vi "Actor Core.vi"(8 "error in":errorcluster, 11 "Nested in":refnum<class "User Interface.lvclass">) -> (0 "error out":errorcluster, 3 "Actor out":refnum<class "Actor.lvclass">)   [LabVIEW 2022 SP3, in "User Interface.lvlib" / "User Interface.lvclass"]
doc: "(<B>Filename</B>: Actor Framework.lvlib:Actor.lvclass:Actor Core.vi)\n\nReceives messages to the actor, reacts to them, and initiates any error handling that may shut the actor down.\n\nDescendant classes may override this VI to append parallel tasks for the actor to complete while it handles messages. Overrides use the Call Parent Method node."
uses:
  User Interface.lvclass
  C:/Program Files/National Instruments/LabVIEW 2022/vi.lib/ActorFramework/Actor/Actor.lvclass
  <vilib>/ActorFramework/Actor/Actor.lvclass
  Typedefs/UI Helper Loop States.ctl
  User Interface.lvclass/User Interface.ctl
  <vilib>/ActorFramework/Actor/Actor.lvclass/Actor.ctl
  <vilib>/ActorFramework/Message Enqueuer/Message Enqueuer.lvclass/Message Enqueuer.ctl
  User Interface Messages/Update Status String Msg/Update Status String Msg.lvclass/Update Status String Msg.ctl
  User Interface Messages/Stop Test using Abs Msg/Stop Test using Abs Msg.lvclass/Stop Test using Abs Msg.ctl
  User Interface Messages/Generate Report Event using Abs Msg/Generate Report Event using Abs Msg.lvclass/Generate Report Event using Abs Msg.ctl
  <vilib>/Utility/miscctls.llb/LVRowAndColumnTypeDef.ctl
  User Interface Messages/Send Abs Start Test Msg/Start Test using Abs Msg.lvclass/Start Test using Abs Msg.ctl
  <vilib>/ActorFramework/Message Enqueuer/Init from Existing Queue.vi
  <vilib>/ActorFramework/Message Enqueuer/Enqueue.vi
  User Interface Messages/Close Application using Abs Msg/Close Application using Abs Msg.lvclass
  C:/Program Files/National Instruments/LabVIEW 2022/vi.lib/ActorFramework/Message/Message.lvclass
  User Interface Messages/Update Status String Msg/Update Status String Msg.lvclass
  User Interface Messages/Stop Test using Abs Msg/Stop Test using Abs Msg.lvclass
  User Interface Messages/Generate Report Event using Abs Msg/Generate Report Event using Abs Msg.lvclass
  User Interface Messages/Send Abs Start Test Msg/Start Test using Abs Msg.lvclass
  <vilib>/ActorFramework/Message Priority Queue/Priority Enqueue.vi
  <vilib>/ActorFramework/Message Enqueuer/Message Enqueuer.lvclass
  User Interface.lvlib
panel:
  in  "Logout":bool
  out "Machine":string
  out "User":string
  in  "Help":bool
  in  "Tab Control":enum32{"Test Execution", "Test Configuration"}(tab)
  in  "Load Selection":bool
  in  "Save Selection":bool
  in  "Overall Result":string
  in  "Print Report":bool
  in  "Stop Test":bool
  in  "Start Test":bool
  in  "Available Tests":i32[](listbox)
  in  "Test Configuration":T1(tab)
  in  "Ping Test":T2(array[cluster])
  in  "Select Path":path
  in  "Select a byte stream File Path":path
  in  "Select Test(s)":u16(ring)
  in  "Clear Status":bool
  out "Status":string
  # "Test Application v0.0"
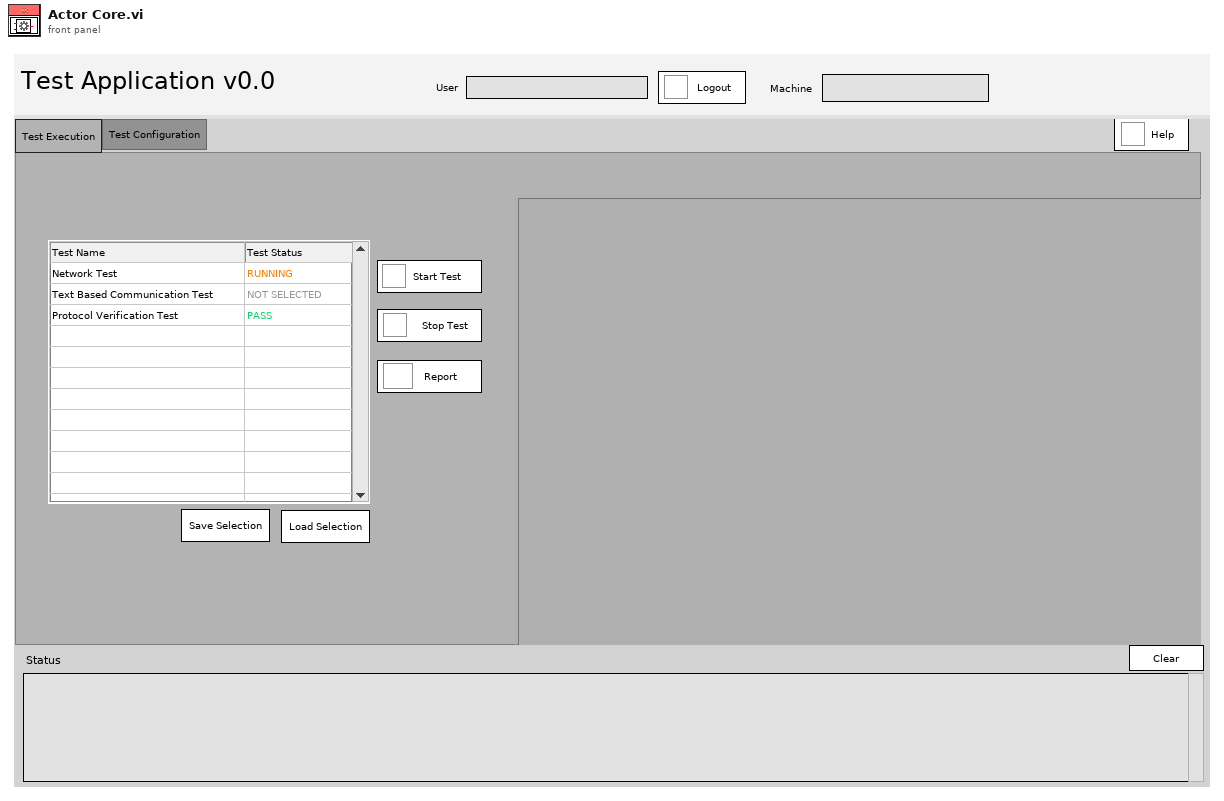
[diagram p1: front panel]
types:
  T1 = enum32{"None", "Network Test", "Text Based Communication Test", "Protocol Verification Test"}
  T2 = cluster{"IP/Address":string, "PacketSize":i32, "timeout":i32, "Packet Count":i32, "Min Expected Packed Return %":dbl, "Ping Result":cluster{"Result?":bool, "Actual Packet Return %":dbl}}[]
  T3 = typedef "User Interface.lvlib/UI Helper Loop States.ctl" = enum16{"Poll", "Init UI", "Load Available Tests", "Start Test", "Error", "Exit"}
  T4 = cluster{"Stop":refnum<user-event>, "Status":refnum<user-event>}
  T5 = enum8{"Enabled", "Disabled", "Disabled and Grayed Out"}
  T6 = typedef "LVRowAndColumnTypeDef.ctl" = cluster{"Row":i32, "Column":i32}
  T7 = typedef "Paths.ctl" = cluster{"Data Directory":path, "Test Config Dir":path, "Error Logs":path, "Event Logs":path, "Settings.Json":path, "Reports Directory":path}
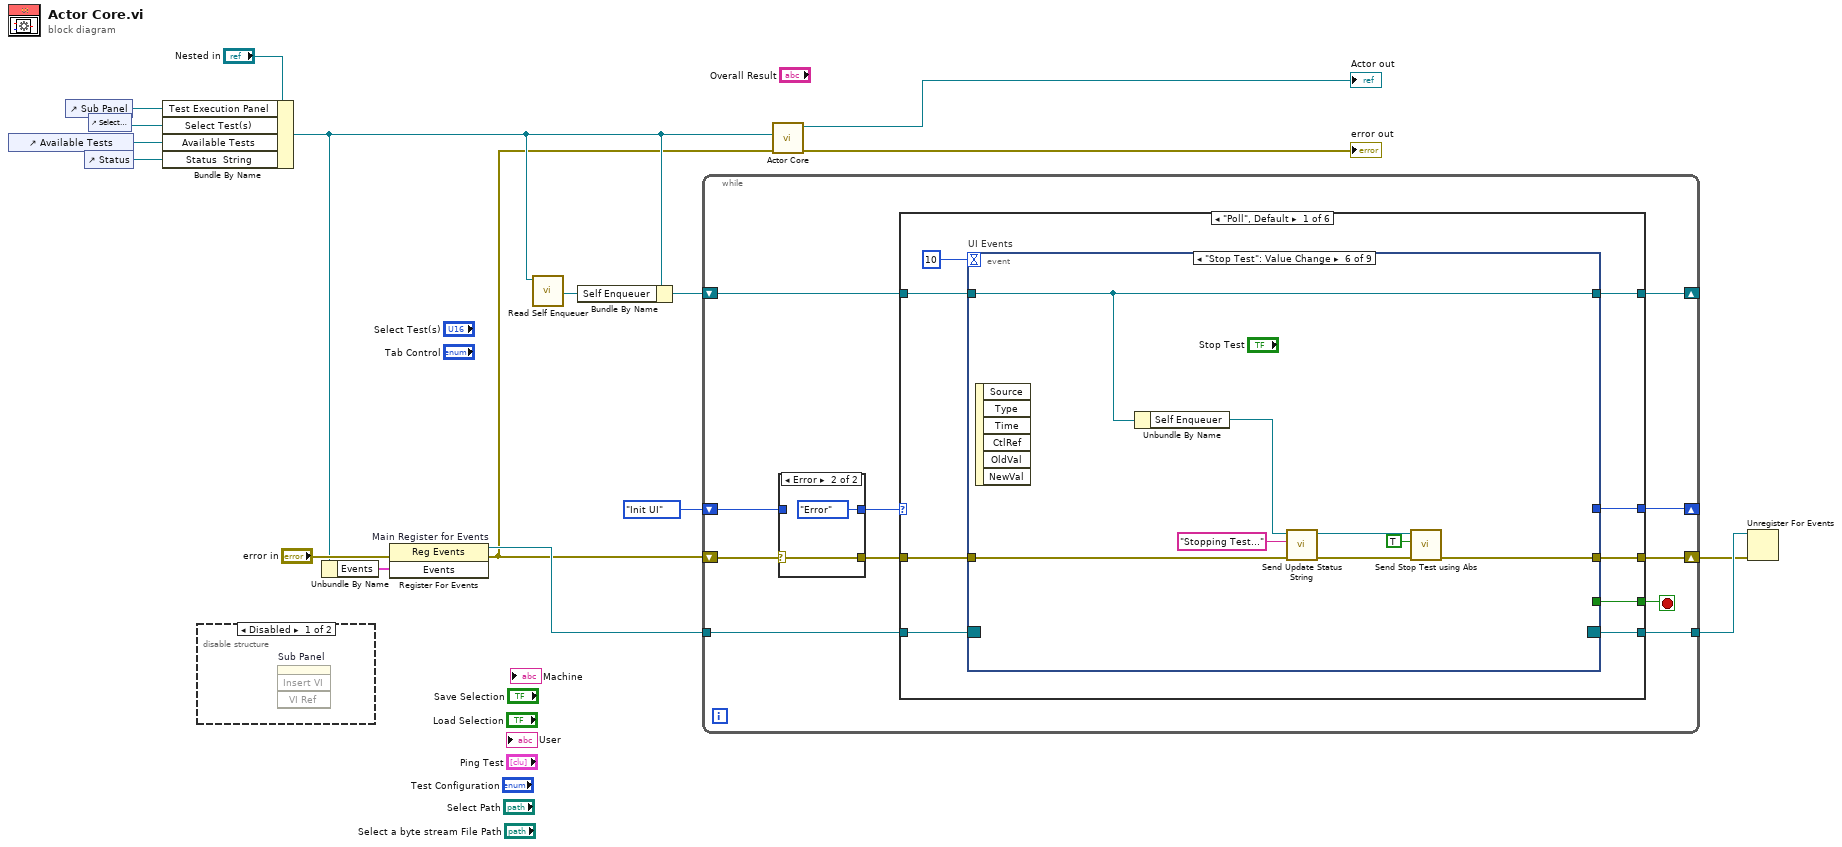
[diagram p0: block diagram]
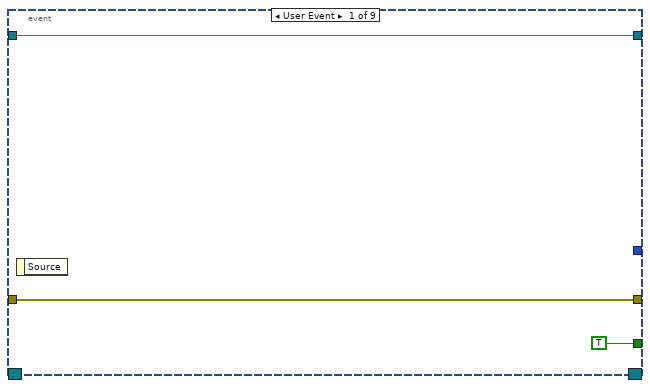
[diagram p4: hidden frame]
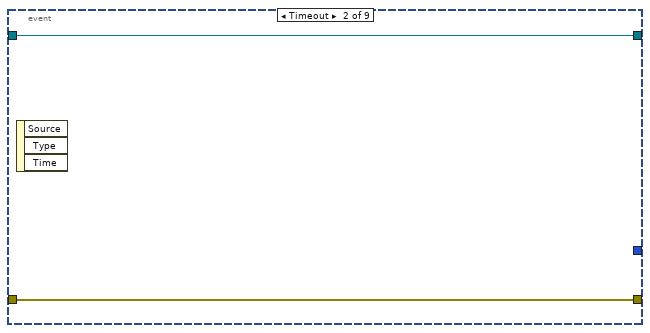
[diagram p5: hidden frame]
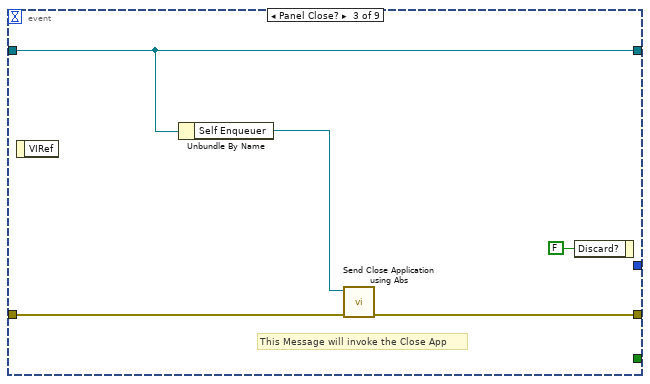
[diagram p6: hidden frame]
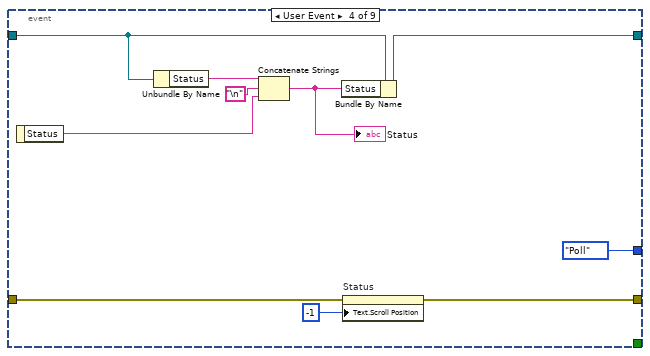
[diagram p7: hidden frame]
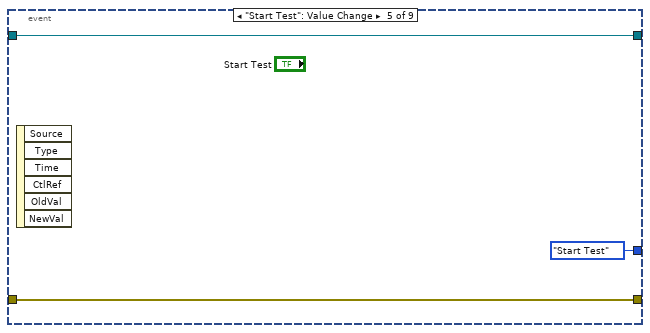
[diagram p8: hidden frame]
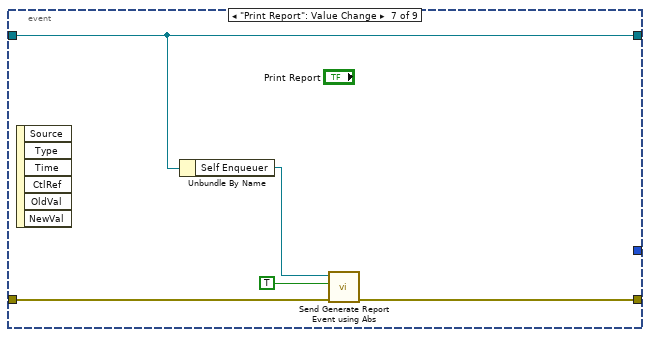
[diagram p9: hidden frame]
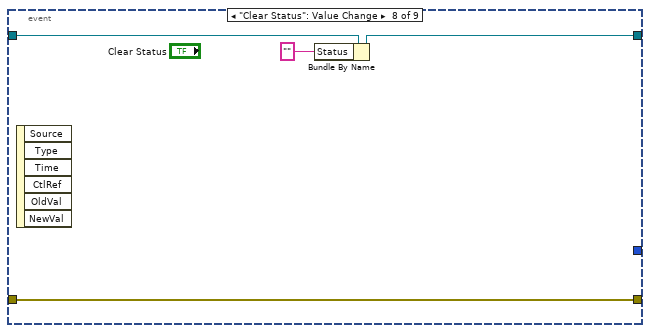
[diagram p10: hidden frame]
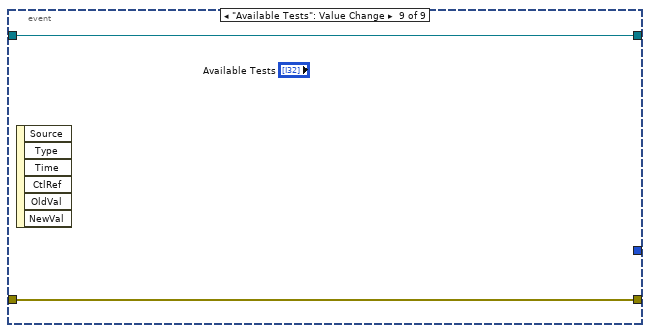
[diagram p11: hidden frame]
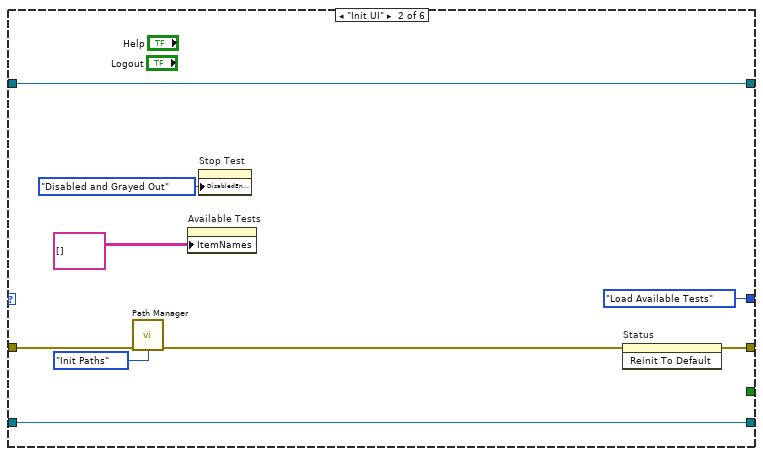
[diagram p12: hidden frame]
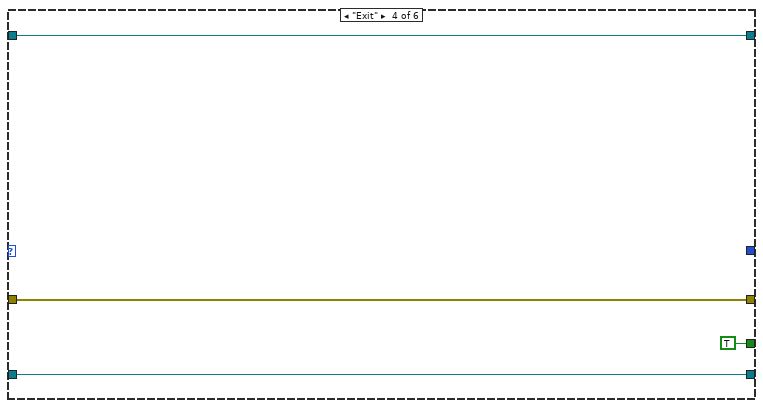
[diagram p14: hidden frame]
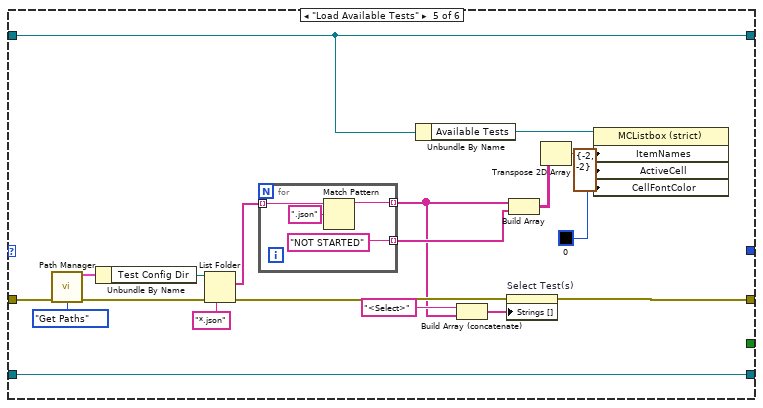
[diagram p15: hidden frame]
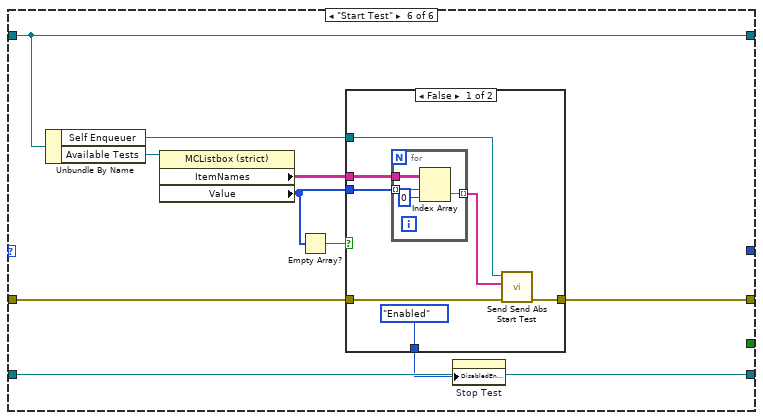
[diagram p16: hidden frame]
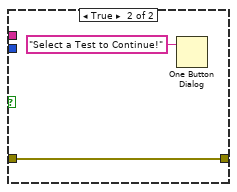
[diagram p17: hidden frame]
diagram:
  n1 = control-ref of="Available Tests"() -> (w6:refnum<vi>)
  n2 = control-ref of="Sub Panel"() -> (w9:refnum<vi>)
  n3 = control-ref of="Status"() -> (w8:refnum<vi>)
  n4 = control-ref of="Select Test(s)"() -> (w7:refnum<vi>)
  n5 = Bundle By Name(cluster="Nested in", "Test Execution Panel"=w9, "Select Test(s)"=w7, "Available Tests"=w6, "Status  String"=w8) -> (w4:refnum<class "User Interface.lvclass">)
  n6 = disable-structure shown="Disabled" {
    frame Disabled {
      n7 = invoke on="Sub Panel" class="SubPnl" method="Insert VI"() -> ()  [unwired: 4 in, 4 out]
    }
    frame Enabled {
    }
  }
  n8 = Unbundle By Name(w4) -> ("Events"=w14:T4)
  n9 = register-events "Main Register for Events"(error in="error in", w14) -> (reference out=w15:refnum<event-registration>, error out=w3:errorcluster)  [unwired: 1 in]
  n10 = call <vilib>:"Read Self Enqueuer.vi"("Actor"=w4) -> ("Self Enqueuer"=w10:refnum<class "Message Enqueuer.lvclass">)  [unwired: 10 in]
  n11 = Bundle By Name(cluster=w4, "Self Enqueuer"=w10) -> (w11:refnum<class "User Interface.lvclass">)
  n12 = while {
    tunnel: w15 -> [w28]
    tunnel: [w26] -> w13
    shift-right: [w24] -> _
    shift-left: w11 -> [w25]
    shift-right: [w23] -> w2
    shift-left: w3 -> [w22]
    shift-right: [w18] -> _
    shift-left: UI_Helper_Loop_States."Init UI" -> [w20]
    stop <- w27 stop-if-true
    n13 = case shown="Error" w22 {
      selector: w22 -> [w30 w31]
      tunnel: [w30 w31] -> w21
      tunnel: w20 -> [w29 _]
      tunnel: [w29 UI_Helper_Loop_States."Error"] -> w19
      frame No Error {
      }
      frame Error {
      }
    }
    n14 = case shown="\"Poll\", Default" w19 {
      tunnel: w28 -> [w41 w92 w95 w99 w119 w133]
      tunnel: [w40 _ _ TRUE _ _] -> w27
      tunnel: [w39 w92 w95 w99 w119 w133] -> w26
      tunnel: w25 -> [w38 w91 w94 w98 w113 w124]
      tunnel: w21 -> [w37 w88 w93 w97 w115 w126]
      tunnel: [w36 w91 w94 w98 w113 w124] -> w24
      tunnel: [w35 w90 w93 w97 w103 w125] -> w23
      tunnel: [w33 UI_Helper_Loop_States."Load Available Tests" _ _ _ _] -> w18
      frame "Poll", Default {
        n15 = event "UI Events" shown="[5] \"Stop Test\": Value Change" {
          selector: w41 -> [_ _ _ _ _ _ _ _ _]
          dyn-events: [_ _ _ _ _ _ _ _ _] -> w39
          timeout: 10 -> [_ _ _ _ _ _ _ _ _]
          tunnel: [TRUE _ _ _ _ _ _ _ _] -> w40
          tunnel: w37 -> [w42 w45 w49 w53 w62 w67 w74 w78 w83]
          tunnel: w38 -> [w43 w46 w50 w61 w64 w72 w77 w81 w82]
          tunnel: [w43 w46 w50 w57 w64 w72 w77 w80 w82] -> w36
          tunnel: [w42 w45 w48 w52 w62 w71 w73 w78 w83] -> w35
          tunnel: [_ _ _ UI_Helper_Loop_States."Poll" UI_Helper_Loop_States."Start Test" _ _ _ _] -> w33
          event User Event {
            n16 = event-data() -> ()  [unwired: 1 in, 1 out]
          }
          event Timeout {
            n17 = event-data() -> ()  [unwired: 1 in, 3 out]
          }
          event Panel Close? {
            # "This Message will invoke the Close App"
            n18 = event-data() -> ()  [unwired: 1 in, 1 out]
            n19 = Unbundle By Name(w50) -> ("Self Enqueuer"=w47:refnum<class "Message Enqueuer.lvclass">)
            n20 = call "Send Close Application using Abs.vi"("error in (no error)"=w49, "Message Enqueuer"=w47) -> ("error out"=w48:errorcluster)  [unwired: 8 in, 1 out]
            n21 = event-data("Discard?"=FALSE) -> ()  [unwired: 1 in, 1 out]
          }
          event User Event {
            n22 = event-data() -> ("Status"=w58:string)  [unwired: 1 in]
            n23 = Unbundle By Name(w61) -> ("Status"=w60:string)
            n24 = Concatenate Strings(w60, "\n", w58) -> (w56:string)
            "Status" <- w56
            n25 = Bundle By Name(cluster=w61, "Status"=w56) -> (w57:refnum<class "User Interface.lvclass">)
            n26 = property on="Status" class="Str"(error in=w53, "Text.Scroll Position"=-1) -> (error out=w52:errorcluster)  [unwired: 1 in, 1 out]
          }
          event "Start Test": Value Change {
            n27 = event-data() -> ()  [unwired: 1 in, 6 out]
          }
          event "Stop Test": Value Change {
            n28 = event-data() -> ()  [unwired: 1 in, 6 out]
            n29 = Unbundle By Name(w72) -> ("Self Enqueuer"=w69:refnum<class "Message Enqueuer.lvclass">)
            n30 = call "Send Update Status String.vi"("error in (no error)"=w67, "Status"="Stopping Test...", "Message Enqueuer"=w69) -> ("error out"=w66:errorcluster, "Message Enqueuer out"=w68:refnum<class "Message Enqueuer.lvclass">)  [unwired: 7 in]
            n31 = call "Send Stop Test using Abs.vi"("error in (no error)"=w66, "Stop Test"=TRUE, "Message Enqueuer"=w68) -> ("error out"=w71:errorcluster)  [unwired: 7 in, 1 out]
          }
          event "Print Report": Value Change {
            n32 = event-data() -> ()  [unwired: 1 in, 6 out]
            n33 = Unbundle By Name(w77) -> ("Self Enqueuer"=w76:refnum<class "Message Enqueuer.lvclass">)
            n34 = call "Send Generate Report Event using Abs.vi"("error in (no error)"=w74, "Generate Report"=TRUE, "Message Enqueuer"=w76) -> ("error out"=w73:errorcluster)  [unwired: 7 in, 1 out]
          }
          event "Clear Status": Value Change {
            n35 = event-data() -> ()  [unwired: 1 in, 6 out]
            n36 = Bundle By Name(cluster=w81, "Status"="") -> (w80:refnum<class "User Interface.lvclass">)
          }
          event "Available Tests": Value Change {
            n37 = event-data() -> ()  [unwired: 1 in, 6 out]
          }
        }
      }
      frame "Init UI" {
        n38 = call "Path Manager.vi"("Error in (no error)"=w88, "Options"=enum16{"Get Paths", "Init Paths"}."Init Paths") -> ("Error out"=w87:errorcluster)  [unwired: 12 in, 1 out]
        n39 = property on="Available Tests" class="MCListbox (strict)"("ItemNames"=string[][] [] ("Item Names")) -> ()  [unwired: 2 in, 2 out]
        n40 = property on="Stop Test" class="Bool"("DisabledEnum"=T5."Disabled and Grayed Out" ("Disabled")) -> ()  [unwired: 2 in, 2 out]
        n41 = invoke on="Status" class="Str" method="Reinit To Default"(error in=w87) -> (error out=w90:errorcluster)  [unwired: 2 in, 2 out]
      }
      frame "Error" {
      }
      frame "Exit" {
      }
      frame "Load Available Tests" {
        n42 = call "Path Manager.vi"("Error in (no error)"=w115, "Options"=enum16{"Get Paths", "Init Paths"}."Get Paths") -> ("Cluster"=w117:T7, "Error out"=w111:errorcluster)  [unwired: 12 in]
        n43 = Unbundle By Name(w117) -> ("Test Config Dir"=w116:path)
        n44 = List Folder(path=w116, pattern="*.json", error in=w111) -> (filenames=w110:string[], error out=w104:errorcluster)  [unwired: 1 in, 2 out]
        n45 = for {
          tunnel: w110 -> [w123] mode=indexing
          tunnel: [w121] -> w101 mode=indexing
          tunnel: ["NOT STARTED"] -> w107 mode=indexing
          n46 = Match Pattern(string=w123, regular expression=".json") -> (before substring=w121:string)  [unwired: 1 in, 3 out]
        }
        n47 = Unbundle By Name(w113) -> ("Available Tests"=w112:refnum<vi>)
        n48 = Build Array (concatenate)("<Select>" ("string"), w101) -> (w100:string[])
        n49 = property on="Select Test(s)" class="Ring (strict)"(error in=w104, "Strings []"=w100) -> (error out=w103:errorcluster)  [unwired: 1 in, 1 out]
        n50 = Build Array(w101, w107) -> (w109:string[][])
        n51 = Transpose 2D Array(2D array=w109) -> (transposed array=w108:string[][])
        n52 = property class="MCListbox (strict)"(reference=w112, "ItemNames"=w108, "ActiveCell"=T6 {"Row"=-2, "Column"=-2} ("Active Cell:Active Cell"), "CellFontColor"=u32 0) -> ()  [unwired: 1 in, 2 out]
      }
      frame "Start Test" {
        n53 = Unbundle By Name(w124) -> ("Self Enqueuer"=w132:refnum<class "Message Enqueuer.lvclass">, "Available Tests"=w131:refnum<vi>)
        n54 = property class="MCListbox (strict)"(reference=w131) -> ("ItemNames"=w130:string[][], "Value"=w129:i32[])  [unwired: 1 in, 2 out]
        n55 = Empty Array?(array=w129) -> (empty?=w128:bool)
        n56 = case shown="False" w128 {
          tunnel: w126 -> [w140 w145]
          tunnel: [w139 w145] -> w125
          tunnel: w132 -> [w138 _]
          tunnel: w130 -> [w137 _]
          tunnel: w129 -> [w136 _]
          tunnel: [T5."Enabled" ("Disabled") _] -> w127
          frame False {
            n57 = for {
              tunnel: w137 -> [w144]
              tunnel: w136 -> [w142] mode=indexing
              tunnel: [w143] -> w135 mode=indexing
              n58 = Index Array(array=w144, index (row)=w142, index (col)=0 ("disabled index (col)")) -> (element=w143:string)
            }
            n59 = call "Send Send Abs Start Test.vi"("error in (no error)"=w140, "Selected Tests"=w135, "Message Enqueuer"=w138) -> ("error out"=w139:errorcluster)  [unwired: 7 in, 1 out]
          }
          frame True {
            n60 = One Button Dialog(message="Select a Test to Continue!") -> ()  [unwired: 1 in, 1 out]
          }
        }
        n61 = property on="Stop Test" class="Bool"("DisabledEnum"=w127) -> ()  [unwired: 2 in, 2 out]
      }
    }
  }
  n62 = call-parent "Actor Core.vi"("error in"=w3, "Actor in"=w4) -> ("error out"=→"error out":errorcluster, "Actor out"=→"Actor out":refnum<class "Actor.lvclass">)  [unwired: 8 in]
  n63 = Unregister For Events(event registration refnum=w13, error in=w2) -> ()  [unwired: 1 out]
